vi "SV_FFT.vi"() -> ()   [LabVIEW 2023]
uses:
  <vilib>/measure/maspectr.llb/Power Spectrum and PSD Export Mode.ctl
  <vilib>/Analysis/4window.llb/windowTd.ctl
  <vilib>/Analysis/2dsp.llb/Real FFT.vi
  <vilib>/measure/maspectr.llb/FFT Power Spectrum and PSD for 1 Chan (CDB).vi
  <vilib>/Utility/file.llb/Read Delimited Spreadsheet (DBL).vi
  <vilib>/gmath/NI_Gmath.lvlib
  <vilib>/Analysis/NI_AALPro.lvlib
  <vilib>/measure/NI_MAPro.lvlib
panel:
  out "LF/HF":dbl
  out "total power":dbl
  out "HF":dbl
  out "LF":dbl
  out "Power Spectrum / PSD":cluster{"f0":dbl, "df":dbl, "magnitude":dbl[]} {"magnitude" format="%.2p"; "f0" format="%0.2p"; "df" format="%0.2p"}
  out "CW_baseline_index":dbl[](array[numeric])
  out "CW_SV_baselinedata":dbl[](array[numeric])
  out "Waveform Graph":cluster{"f0":dbl, "df":dbl, "magnitude":dbl[]}(graph)
  out "SVV baseline inter":cluster{"xi used":dbl[], "yi":dbl[]}(graph)
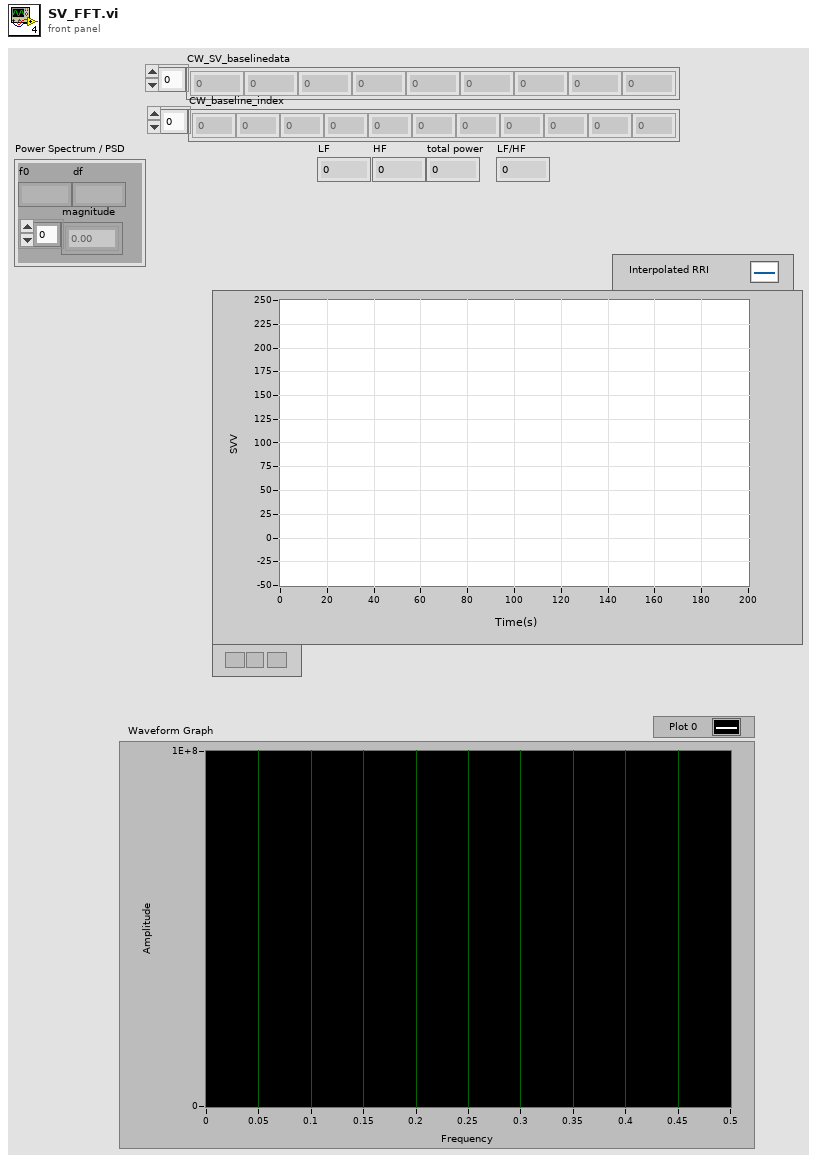
[diagram p1: front panel]
types:
  T1 = typedef "NI_AALPro.lvlib/windowTd.ctl" = u32
  T2 = typedef "NI_MAPro.lvlib/Power Spectrum and PSD Export Mode.ctl" = u16
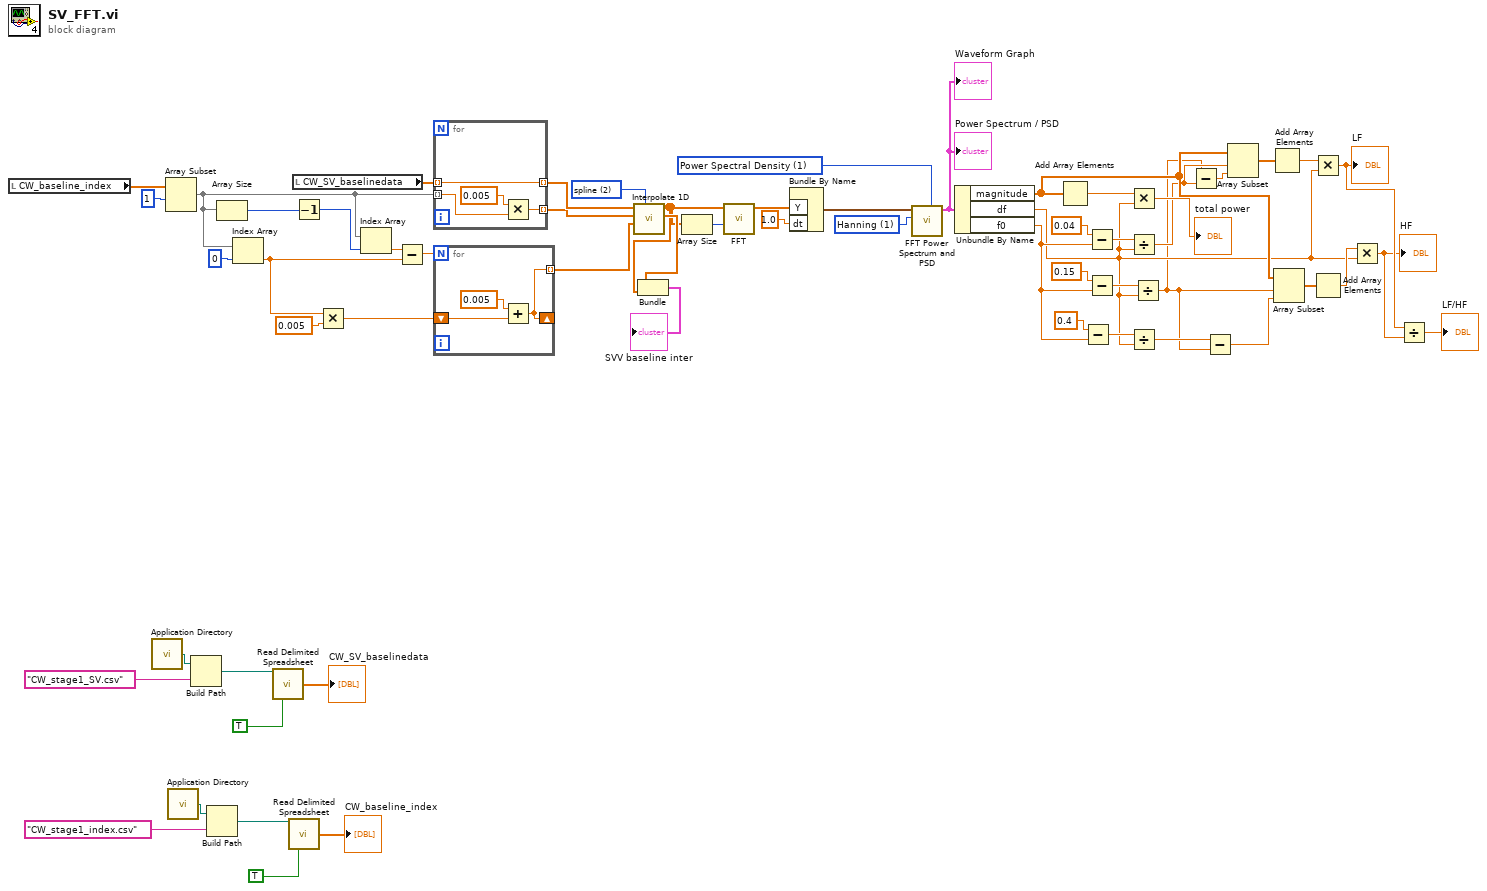
[diagram p0: block diagram]
diagram:
  w35 = T1 1 items=["Rectangle"=0, "Hanning"=1, "Hamming"=2, "Blackman-Harris"=3, "Exact Blackman"=4, "Blackman"=5, "Flat Top"=6, "4 Term B-Harris "=7, "7 Term B-Harris"=8, "Low Sidelobe"=9, "Blackman Nuttall"=11, "Triangle"=30, "Bartlett-Hanning"=31, "Bohman"=32, "Parzen"=33, "Welch"=34, "Kaiser"=60, "Dolph-Chebyshev"=61, "Gaussian"=62] ("window")
  w36 = T2 1 items=["Power Spectrum", "Power Spectral Density"] ("export mode")
  w57 = 2 items=["nearest", "linear", "spline", "cubic Hermite", "Lagrange"] ("method")
  n1 = local read "CW_baseline_index"() -> (w44:dbl[])
  n2 = call <vilib>:"Application Directory.vi"() -> ("Application Directory"=w34:path)
  n3 = Array Subset(array=w44, index=1) -> (w49:dbl[])  [unwired: 1 in]
  n4 = call <vilib>:"Application Directory.vi"() -> ("Application Directory"=w29:path)
  n5 = Build Path(base path=w34, name or relative path="CW_stage1_SV.csv") -> (appended path=w31:path)
  n6 = Build Path(base path=w29, name or relative path="CW_stage1_index.csv") -> (appended path=w26:path)
  n7 = Array Size(array=w49) -> (size(s)=w47:i32)
  n8 = Index Array(array=w49, index=0) -> (element=w53:dbl)
  n9 = call-poly <vilib>:"Read Delimited Spreadsheet.vi"("file path (dialog if empty)"=w31, "transpose? (F)"=TRUE) -> ("first row"=→"CW_SV_baselinedata":dbl[])  [unwired: 8 in, 5 out]
  n10 = call-poly <vilib>:"Read Delimited Spreadsheet.vi"("file path (dialog if empty)"=w26, "transpose? (F)"=TRUE) -> ("first row"=→"CW_baseline_index":dbl[])  [unwired: 8 in, 5 out]
  n11 = local read "CW_SV_baselinedata"() -> (w42:dbl[])
  n12 = Decrement(x=w47) -> (x-1=w48:i32)
  n13 = Multiply(x=w53, y=0.005) -> (x*y=w55:dbl)
  n14 = Index Array(array=w49, index=w48) -> (element=w51:dbl)
  n15 = Subtract(x=w51, y=w53) -> (x-y=w52:dbl)
  n16 = for {
    tunnel: w42 -> [w60] mode=indexing
    tunnel: w49 -> [w63] mode=indexing
    tunnel: [w61] -> w45 mode=indexing
    tunnel: [w60] -> w46 mode=indexing
    n17 = Multiply(x=0.005, y=w63) -> (x*y=w61:dbl)
  }
  n18 = for {
    N: w52 -> [_]
    shift-right: [w64] -> _
    shift-left: w55 -> [w66]
    tunnel: [w64] -> w56 mode=indexing
    n19 = Add(x=0.005, y=w66) -> (x+y=w64:dbl)
  }
  n20 = call <vilib>:"Interpolate 1D.vi"("method"=w57, "xi"=w56, "X"=w45, "Y"=w46) -> ("xi used"=w58:dbl[], "yi"=w40:dbl[])  [unwired: 5 in, 1 out]
  n21 = Bundle("xi used"=w58, "yi"=w40) -> (→"SVV baseline inter":cluster{"xi used":dbl[], "yi":dbl[]})  [unwired: 1 in]
  n22 = Array Size(array=w40) -> (size(s)=w41:i32)
  n23 = call-poly <vilib>:"FFT.vi"("FFT size"=w41, "X"=w40) -> ("FFT {X}"=w39:cdb[])  [unwired: 8 in, 1 out]
  n24 = Bundle By Name("Y"=w39, "dt"=1.0) -> (w37:waveform(cdb))  [unwired: 1 in]
  n25 = call-poly <vilib>:"FFT Power Spectrum and PSD.vi"("export mode"=w36, "window"=w35, "time signal"=w37) -> ("Power Spectrum / PSD"=w24:cluster{"f0":dbl, "df":dbl, "magnitude":dbl[]})  [unwired: 5 in, 3 out]
  "Waveform Graph" <- w24
  "Power Spectrum / PSD" <- w24
  n26 = Unbundle By Name(w24) -> ("magnitude"=w9:dbl[], "df"=w7:dbl, "f0"=w15:dbl)
  n27 = Add Array Elements(numeric array=w9) -> (sum=w8:dbl)
  n28 = Subtract(x=0.4, y=w15) -> (x-y=w14:dbl)
  n29 = Subtract(x=0.04, y=w15) -> (x-y=w19:dbl)
  n30 = Subtract(x=0.15, y=w15) -> (x-y=w17:dbl)
  n31 = Multiply(x=w8, y=w7) -> (x*y=→"total power":dbl)
  n32 = Divide(x=w19, y=w7) -> (x/y=w5:dbl)
  n33 = Divide(x=w14, y=w7) -> (x/y=w13:dbl)
  n34 = Divide(x=w17, y=w7) -> (x/y=w4:dbl)
  n35 = Subtract(x=w4, y=w5) -> (x-y=w23:dbl)
  n36 = Subtract(x=w13, y=w4) -> (x-y=w12:dbl)
  n37 = Array Subset(array=w9, index=w5, length=w23) -> (w22:dbl[])
  n38 = Add Array Elements(numeric array=w22) -> (sum=w21:dbl)
  n39 = Array Subset(array=w9, index=w4, length=w12) -> (w11:dbl[])
  n40 = Multiply(x=w21, y=w7) -> (x*y=w3:dbl)
  "LF" <- w3
  n41 = Add Array Elements(numeric array=w11) -> (sum=w10:dbl)
  n42 = Multiply(x=w10, y=w7) -> (x*y=w2:dbl)
  "HF" <- w2
  n43 = Divide(x=w3, y=w2) -> (x/y=→"LF/HF":dbl)
